vi "Escritura del Com.vi"(8 "error in (no error)":errorcluster, 10 "write buffer":string, 11 "VISA Refnum in":refnum<visa-resource-name>) -> (0 "error out":errorcluster, 3 "VISA resource name out":refnum<visa-resource-name>)   [LabVIEW 2019, in "Serial Devices.lvlib"]
uses:
  Serial Devices.lvlib
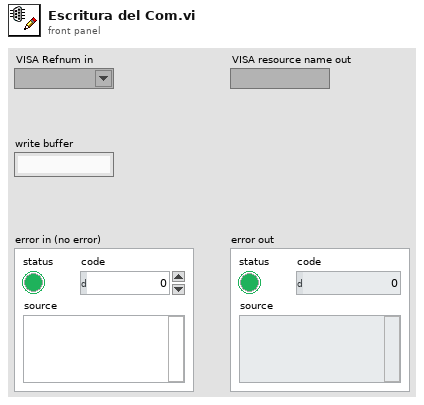
[diagram p1: front panel]
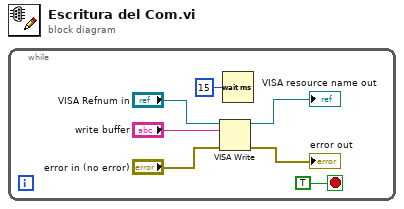
[diagram p0: block diagram]
diagram:
  n1 = while {
    stop <- TRUE stop-if-true
    n2 = VISA Write(VISA resource name="VISA Refnum in", write buffer="write buffer", error in (no error)="error in (no error)") -> (VISA resource name out=→"VISA resource name out":refnum<visa-resource-name>, error out=→"error out":errorcluster)  [unwired: 1 out]
    n3 = Wait (ms)(milliseconds to wait=u32 15) -> ()  [unwired: 1 out]
  }
